vi "RageErrorCodes.vi"(8 "error in":errorcluster) -> (0 "error out":errorcluster, 2 "desc ary":string[](array[string]), 5 "Desc.":string)   [LabVIEW 2018]
uses:
  <vilib>/Utility/file.llb/Read Delimited Spreadsheet (string).vi
panel:
  in  "file path (dialog if empty)":path=path "C:/RageATE/Infrastructure/RageErrorCodes.csv"
  out "all rows":string[][](array[string])
  # "Input a code and error \nMake sure there is a matching code in the Rage file"
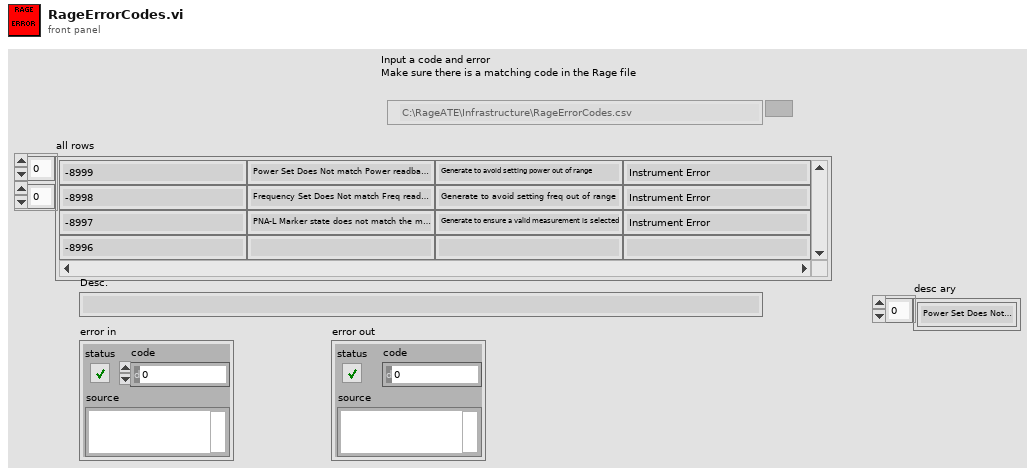
[diagram p1: front panel]
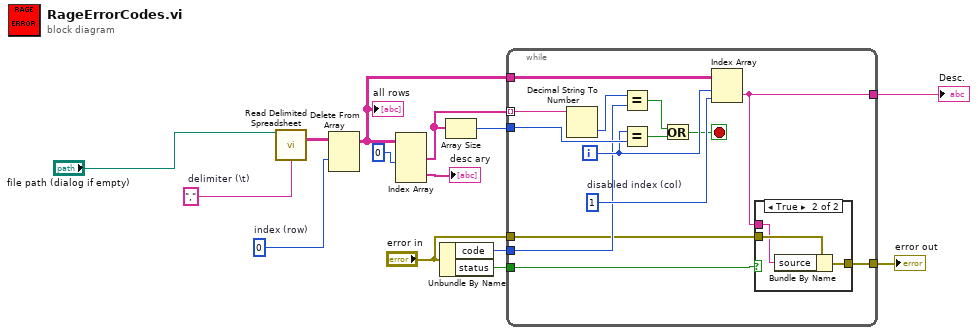
[diagram p0: block diagram]
diagram:
  w8 = 0  # index (row)
  w13 = ","  # delimiter (\t)
  n1 = call-poly <vilib>:"Read Delimited Spreadsheet.vi"("file path (dialog if empty)"="file path (dialog if empty)", "delimiter (\\t)"=w13) -> ("all rows"=w7:string[][])  [unwired: 8 in, 5 out]
  n2 = Delete From Array(array=w7, index (row)=w8) -> (array with subset deleted=w6:string[][])  [unwired: 2 in, 1 out]
  "all rows" <- w6
  n3 = Index Array(array=w6, index (col) #1=0 ("disabled index (col)")) -> (element #1=w4:string[], element #2=→"desc ary":string[])  [unwired: 3 in]
  n4 = Unbundle By Name("error in") -> ("code"=w3:i32, "status"=w2:bool)
  n5 = Array Size(array=w4) -> (size(s)=w11:i32)
  n6 = while {
    tunnel: w4 -> [w27] mode=indexing
    tunnel: w3 -> [w21]
    tunnel: w11 -> [w26]
    tunnel: w6 -> [w25]
    tunnel: [w15] -> w10
    tunnel: [w17] -> w9
    tunnel: w2 -> [w18]
    tunnel: "error in" -> [w16]
    i -> [w24]
    stop <- w20 stop-if-true
    w23 = 1  # disabled index (col)
    n7 = Decimal String To Number(string=w27) -> (number=w28:i32)  [unwired: 2 in, 1 out]
    n8 = Equal?(x=w28, y=w21) -> (x = y?=w19:bool)
    n9 = Equal?(x=w24, y=w26) -> (x = y?=w22:bool)
    n10 = Or(x=w19, y=w22) -> (x .or. y?=w20:bool)
    n11 = Index Array(array=w25, index (row)=w24, index (col)=w23) -> (element=w15:string)
    n12 = case shown="True" w18 {
      tunnel: [w29 w32] -> w17
      tunnel: w16 -> [w29 w31]
      tunnel: w15 -> [_ w30]
      frame False {
      }
      frame True {
        n13 = Bundle By Name(cluster=w31, "source"=w30) -> (w32:errorcluster)
      }
    }
  }
  "Desc." <- w10
  "error out" <- w9
